vi "Serial Comms.vi"(11 "Enum":T1) -> ()   [LabVIEW 2014]
uses:
  TypeDefs/SRE Enum.ctl
panel:
  in  "To Write":string
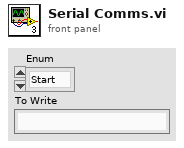
[diagram p1: front panel]
types:
  T1 = typedef "SRE Enum.ctl" = enum16{"Start", "Run", "End"}
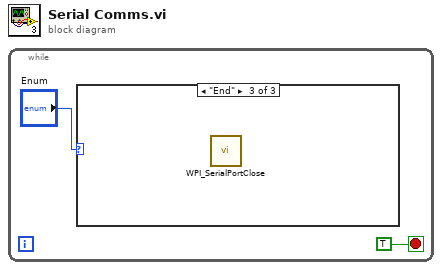
[diagram p0: block diagram]
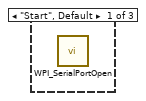
[diagram p2: hidden frame]
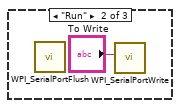
[diagram p3: hidden frame]
diagram:
  n1 = while {
    stop <- TRUE stop-if-true
    n2 = case shown="\"End\"" "Enum" {
      frame "Start", Default {
        n3 = call <vilib>:"WPI_SerialPortOpen.vi"() -> ()  [unwired: 14 in, 2 out]
      }
      frame "Run" {
        n4 = call <vilib>:"WPI_SerialPortFlush.vi"() -> ()  [unwired: 10 in, 2 out]
        n5 = call <vilib>:"WPI_SerialPortWrite.vi"("Buffer"="To Write") -> ()  [unwired: 8 in, 3 out]
      }
      frame "End" {
        n6 = call <vilib>:"WPI_SerialPortClose.vi"() -> ()  [unwired: 11 in, 1 out]
      }
    }
  }
